vi "Get Item Data.vi"(8 "error in (no error)":errorcluster, 11 "VI in":refnum<class "VI.lvclass">) -> (0 "error out":errorcluster, 3 "VI out":refnum<class "VI.lvclass">)   [LabVIEW 2020, in "VI Properties Editor.lvlib" / "VI.lvclass"]
doc: "Gets the info of <B>VI in</B>."
uses:
  VI.lvclass
  C:/Users/acasalen/Documents/LabVIEW Data/Projects/VI-Properties-Editor/source/Classes/Item/Item.lvclass
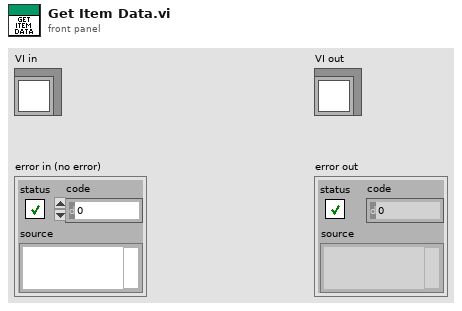
[diagram p1: front panel]
types:
  T1 = enum32{"invalid VI type", "Standard VI", "Control VI", "Global VI", "Polymorphic VI", "Configuration VI", "SubSystem", "Facade VI", "Method VI", "Statechart Diagram VI"}
  T2 = typedef "imagedata.ctl" = cluster{"image type":i32, "image depth":i32, "image":u8[], "mask":u8[], "colors":u32[], "Rectangle":cluster{"left":i16, "top":i16, "right":i16, "bottom":i16}}
  T3 = enum16{"Share clones between instances", "Preallocate clone for each instance"}
  T4 = enum32{"invalid priority", "background priority", "normal priority", "above normal priority", "high priority", "time critical priority", "subroutine"}
  T5 = enum32{"invalid execution system", "user interface", "standard", "instrument i/o", "data acquisition", "other 1", "other 2", "same as caller"}
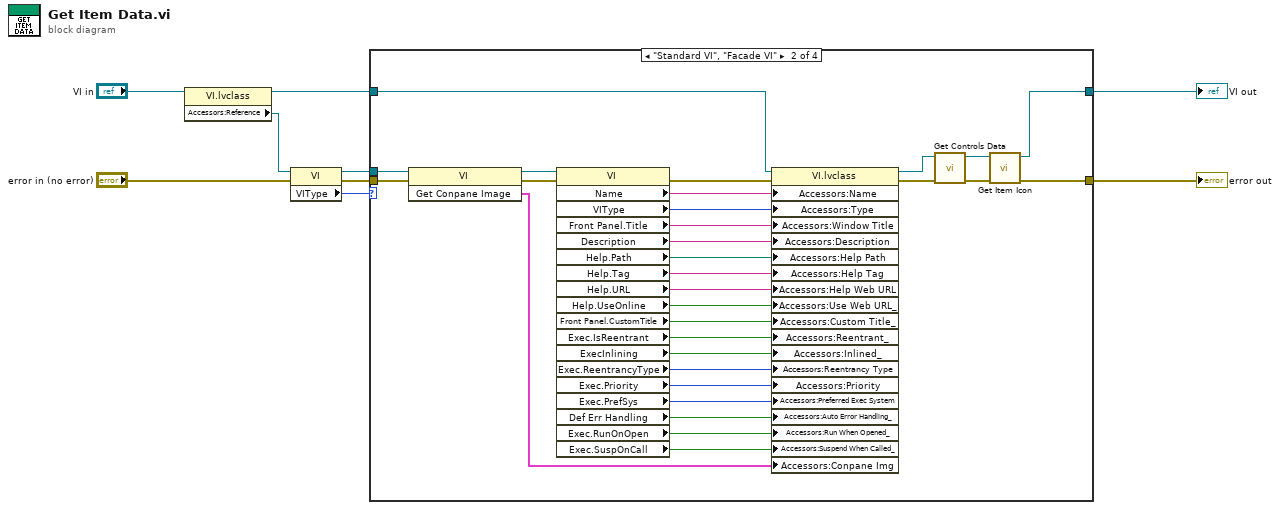
[diagram p0: block diagram]
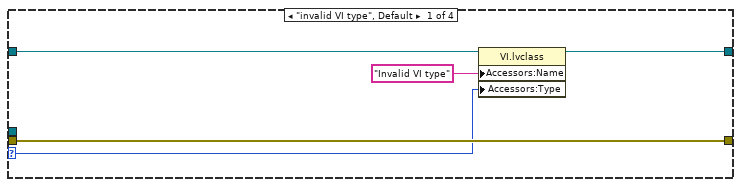
[diagram p2: hidden frame]
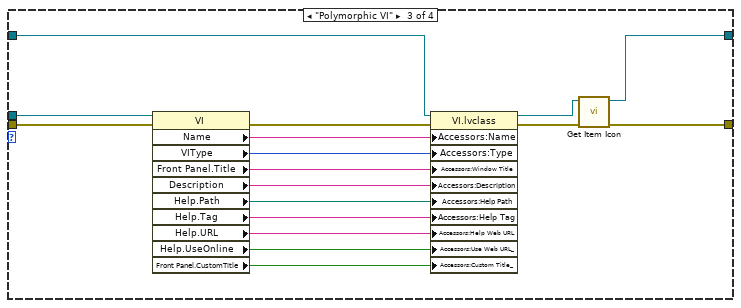
[diagram p3: hidden frame]
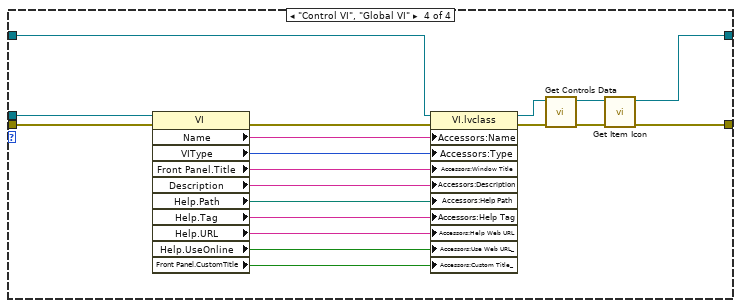
[diagram p4: hidden frame]
diagram:
  n1 = property class="VI.lvclass"(reference="VI in") -> (reference out=w5:refnum<class "VI.lvclass">, "Accessors:Reference"=w6:refnum<vi>)  [unwired: 1 in, 1 out]
  n2 = property class="VI"(reference=w6, error in="error in (no error)") -> (reference out=w2:refnum<vi>, error out=w9:errorcluster, "VIType"=w8:T1)
  n3 = case shown="\"Standard VI\", \"Facade VI\"" w8 {
    selector: w8 -> [w10 _ _ _]
    tunnel: w9 -> [w14 w44 w60 w79]
    tunnel: [w14 w16 w45 w63] -> w3
    tunnel: w5 -> [w13 w42 w58 w77]
    tunnel: [w11 w15 w46 w62] -> w4
    tunnel: w2 -> [_ w21 w61 w80]
    frame "invalid VI type", Default {
      # "Information to path for invalid VI"
      n4 = property class="VI.lvclass"(reference=w13, "Accessors:Name"="Invalid VI type" ("Help.Tag"), "Accessors:Type"=w10) -> (reference out=w11:refnum<class "VI.lvclass">)  [unwired: 1 in, 1 out]
    }
    frame "Standard VI", "Facade VI" {
      n5 = invoke class="VI" method="Get Conpane Image"(reference=w21, error in=w44) -> (reference out=w20:refnum<vi>, error out=w22:errorcluster, "Get Conpane Image"=w19:T2)  [unwired: 1 in]
      n6 = property class="VI"(reference=w20, error in=w22) -> (error out=w43:errorcluster, "Name"=w39:string, "VIType"=w38:T1, "Front Panel.Title"=w37:string, "Description"=w36:string, "Help.Path"=w35:path, "Help.Tag"=w34:string, "Help.URL"=w33:string, "Help.UseOnline"=w32:bool, "Front Panel.CustomTitle"=w31:bool, "Exec.IsReentrant"=w30:bool, "ExecInlining"=w29:bool, "Exec.ReentrancyType"=w28:T3, "Exec.Priority"=w27:T4, "Exec.PrefSys"=w26:T5, "Def Err Handling"=w25:bool, "Exec.RunOnOpen"=w24:bool, "Exec.SuspOnCall"=w23:bool)  [unwired: 1 out]
      n7 = property class="VI.lvclass"(reference=w42, error in=w43, "Accessors:Name"=w39, "Accessors:Type"=w38, "Accessors:Window Title"=w37, "Accessors:Description"=w36, "Accessors:Help Path"=w35, "Accessors:Help Tag"=w34, "Accessors:Help Web URL"=w33, "Accessors:Use Web URL_"=w32, "Accessors:Custom Title_"=w31, "Accessors:Reentrant_"=w30, "Accessors:Inlined_"=w29, "Accessors:Reentrancy Type"=w28, "Accessors:Priority"=w27, "Accessors:Preferred Exec System"=w26, "Accessors:Auto Error Handling_"=w25, "Accessors:Run When Opened_"=w24, "Accessors:Suspend When Called_"=w23, "Accessors:Conpane Img"=w19) -> (reference out=w40:refnum<class "VI.lvclass">, error out=w41:errorcluster)
      n8 = call-dynamic "Get Controls Data.vi"("error in (no error)"=w41, "VI in"=w40) -> ("error out"=w18:errorcluster, "VI out"=w17:refnum<class "VI.lvclass">)  [unwired: 8 in]
      n9 = call-dynamic "Get Item Icon.vi"("error in (no error)"=w18, "VI in"=w17) -> ("error out"=w16:errorcluster, "VI out"=w15:refnum<class "VI.lvclass">)  [unwired: 8 in]
    }
    frame "Polymorphic VI" {
      n10 = property class="VI"(reference=w61, error in=w60) -> (error out=w59:errorcluster, "Name"=w57:string, "VIType"=w56:T1, "Front Panel.Title"=w55:string, "Description"=w54:string, "Help.Path"=w53:path, "Help.Tag"=w52:string, "Help.URL"=w51:string, "Help.UseOnline"=w50:bool, "Front Panel.CustomTitle"=w49:bool)  [unwired: 1 out]
      n11 = property class="VI.lvclass"(reference=w58, error in=w59, "Accessors:Name"=w57, "Accessors:Type"=w56, "Accessors:Window Title"=w55, "Accessors:Description"=w54, "Accessors:Help Path"=w53, "Accessors:Help Tag"=w52, "Accessors:Help Web URL"=w51, "Accessors:Use Web URL_"=w50, "Accessors:Custom Title_"=w49) -> (reference out=w47:refnum<class "VI.lvclass">, error out=w48:errorcluster)
      n12 = call-dynamic "Get Item Icon.vi"("error in (no error)"=w48, "VI in"=w47) -> ("error out"=w45:errorcluster, "VI out"=w46:refnum<class "VI.lvclass">)  [unwired: 8 in]
    }
    frame "Control VI", "Global VI" {
      n13 = property class="VI"(reference=w80, error in=w79) -> (error out=w78:errorcluster, "Name"=w76:string, "VIType"=w75:T1, "Front Panel.Title"=w74:string, "Description"=w73:string, "Help.Path"=w72:path, "Help.Tag"=w71:string, "Help.URL"=w70:string, "Help.UseOnline"=w69:bool, "Front Panel.CustomTitle"=w68:bool)  [unwired: 1 out]
      n14 = property class="VI.lvclass"(reference=w77, error in=w78, "Accessors:Name"=w76, "Accessors:Type"=w75, "Accessors:Window Title"=w74, "Accessors:Description"=w73, "Accessors:Help Path"=w72, "Accessors:Help Tag"=w71, "Accessors:Help Web URL"=w70, "Accessors:Use Web URL_"=w69, "Accessors:Custom Title_"=w68) -> (reference out=w66:refnum<class "VI.lvclass">, error out=w67:errorcluster)
      n15 = call-dynamic "Get Controls Data.vi"("error in (no error)"=w67, "VI in"=w66) -> ("error out"=w65:errorcluster, "VI out"=w64:refnum<class "VI.lvclass">)  [unwired: 8 in]
      n16 = call-dynamic "Get Item Icon.vi"("error in (no error)"=w65, "VI in"=w64) -> ("error out"=w63:errorcluster, "VI out"=w62:refnum<class "VI.lvclass">)  [unwired: 8 in]
    }
  }
  "error out" <- w3
  "VI out" <- w4
